vi "Dashboard Main.vi"() -> ()   [LabVIEW 2018]
uses:
  <vilib>/Rock Robotics/WPI/Camera/WPI_CameraExposure Values.ctl
  <vilib>/Rock Robotics/WPI/Camera/WPI_CameraWhite Balance Values.ctl
  <vilib>/Rock Robotics/WPI/Camera/WPI_CameraSettings Read MJPG.ctl
  <vilib>/Rock Robotics/WPI/Camera/WPI_CameraImageSize.ctl
  <vilib>/Utility/miscctls.llb/LVRowAndColumnTypeDef.ctl
  <vilib>/event_ctls.llb/eventvkey.ctl
  <vilib>/Rock Robotics/Network Tables/NT Read Numeric Array.vi
  <vilib>/Rock Robotics/WPI/Dashboard/WPI_DashboardLogging Global.vi
  Dashboard globals.vi
  <vilib>/vision/NI_Vision_Development_Module.lvlib
panel:
  in  "Camera Settings Right":T1={"Frame Rate"=30, "Compression"=30, "Size"=1, "DB Camera Config"=FALSE} {"Frame Rate" scale=1.0..30.0; "Compression" scale=100.0..-1.0; "Size" items=["640x480", "320x240", "160x120"]}
  in  "Camera Name Right":string(combo)="No Camera Selection"
  out "Camera Perf":string
  in  "Camera Settings":T1={"Frame Rate"=30, "Compression"=30, "Size"=1, "DB Camera Config"=FALSE} {"Frame Rate" scale=1.0..30.0; "Compression" scale=100.0..-1.0; "Size" items=["640x480", "320x240", "160x120"]}
  in  "TCP":refnum<k5>
  in  "Rec Mode":enum32{"Stop", "Record", "Playback"}(radio)
  out "Robot IP":string
  out "Image Message":string="Timeout in Camera Communications"
  in  "Dashboard Tab":T2(tab)=enum."Custom"
  in  "Select Auto":string(combo)="Select Autonomous ..."
  out "NT Connection":bool
  out "MotorChart R":cluster{"Numeric":dbl, "Numeric":dbl}(graph)
  out "MotorChart L":cluster{"Numeric":dbl, "Numeric":dbl}(graph)
  out "MotorSliders R":cluster{"MotorSlide1":dbl, "MotorSlide2":dbl} {"MotorSlide2" scale=-1.0..1.0 scale format="%#_2e"; "MotorSlide1" scale=-1.0..1.0 scale format="%#_2e"}
  out "MotorSliders L":cluster{"MotorSlide1":dbl, "MotorSlide2":dbl} {"MotorSlide2" scale=-1.0..1.0 scale format="%#_2e"; "MotorSlide1" scale=-1.0..1.0 scale format="%#_2e"}
  out "Gyro":dbl(knob) scale=0.0..360.0
  out "JS1 Z":dbl(slide) scale=-1.0..1.0 scale format="%#_2e"
  out "JS1 Graph":cluster{"X":dbl, "Y":dbl}[](graph)
  out "JS1 Buttons":T3
  out "JS2 Z":dbl(slide) scale=-1.0..1.0 scale format="%#_2e"
  out "JS2 Graph":cluster{"X":dbl, "Y":dbl}[](graph)
  out "JS2 Buttons":T3
  out "Mode":T4(ring)=enum."Auto Disabled"
  out "Right Camera Perf":cluster{"Bandwidth (Mbps)":dbl, "FPS":dbl}
  out "Camera Image Right":T5(plugin-control)
  in  "DB/String 9":string
  in  "DB/String 8":string
  in  "DB/String 7":string
  in  "DB/String 6":string
  in  "DB/String 5":string
  in  "DB/String 4":string
  in  "DB/String 3":string
  in  "DB/String 2":string
  in  "DB/String 1":string
  in  "DB/String 0":string
  in  "DB/Slider 0":dbl(slide) scale=0.0..5.0
  in  "DB/Slider 1":dbl(slide) scale=0.0..5.0
  in  "DB/Slider 2":dbl(slide) scale=0.0..5.0
  in  "DB/Slider 3":dbl(slide) scale=0.0..5.0
  out "DB/LED 3":bool
  out "DB/LED 2":bool
  out "DB/LED 1":bool
  out "DB/LED 0":bool
  in  "DB/Button 3":bool
  in  "DB/Button 2":bool
  in  "DB/Button 1":bool
  in  "DB/Button 0":bool caption="New Name"
  in  "Desired Target":T6(radio)=enum."Ship Right"
  in  "Enable Vision\nProcessing":bool
  in  "Test Slider":dbl(slide) scale=0.0..100.0 scale format="%#_3g"
  in  "On/Off":bool caption="Solenoid"
  in  "Test Name":u16(ring) items=["Select the test to run..."]
  in  "Test Tree":string(tree)
  in  "Motor":cluster{"Value":dbl, "Enable":bool} {"Value" scale=-1.0..1.0 scale format="%#_3g"}
  out "Progress":T7 {"Test Progress" scale=0.0..100.0}
  in  "Rev/Fwd":cluster{"Forward":bool, "Reverse":bool}
  in  "Test Ring":u16(ring) items=["Monochrome", "Color"]
  out "Cmd Status":string
  in  "Execute Command":bool
  in  "Command Params":string[][](table)
  in  "Command Selection":i32(listbox)
  in  "CheckList":i32(listbox)
  out "Tree":string(tree)
  out "Camera Image":T5(plugin-control)
  out "Background":bool
  in  "Camera Name":string(combo)="No Camera Selection"
  # "HW"
  # "HW"
  # "Joysticks"
  # "Drive Motors"
  # "Front"
  # "Right"
  # "Left"
  # "Back"
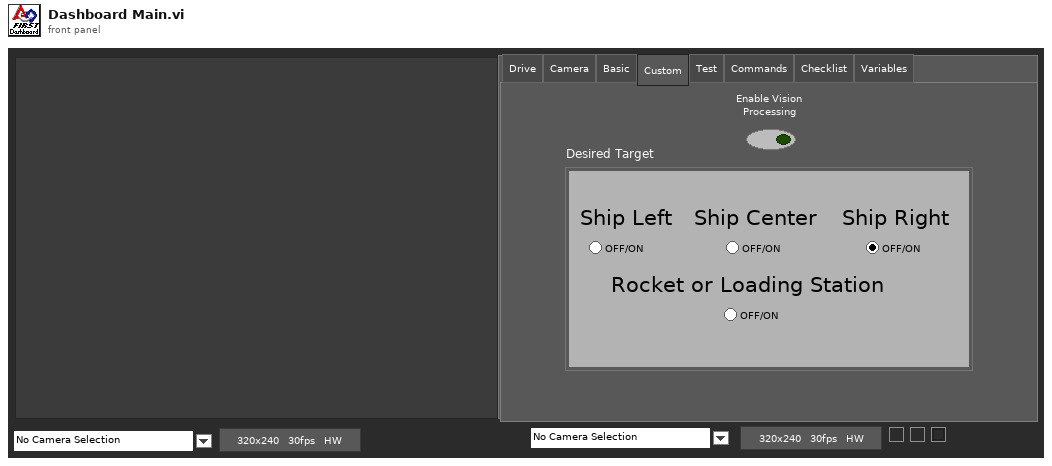
[diagram p1: front panel]
types:
  T1 = cluster{"Frame Rate":i32, "Compression":i32, "Size":u16, "DB Camera Config":bool}
  T2 = enum32{"Drive", "Camera", "Basic", "Custom", "Test", "Commands", "Checklist", "Variables"}
  T3 = cluster{bool, bool, bool, bool, bool, bool, bool, bool, bool, bool, bool, bool}
  T4 = enum8{"Tele-Op Disabled", "Tele-Op Enabled", "Auto Disabled", "Auto Enabled", "Test Disabled", "Test Enabled", "Disconnected", "No Code", "E-Stop"}
  T5 = typedef "IMAQ Image.ctl" = refnum<image>
  T6 = enum32{"Ship Left", "Ship Center", "Ship Right", "Rocket or Loading Station"}
  T7 = cluster{"Test Progress":u8, "Test Progress Text":string}
  T8 = cluster{"Save Path":path, "Interval (s)":dbl, "Keep":i32}
  T9 = typedef "Image Type" = u32
  T10 = cluster{"IDs":cluster{"RPC field ID":u16, "Unique ID":u16}, "String":string}
  T11 = cluster{"Camera Image":refnum<vi>, "Dashboard Tab":refnum<vi>, "Background":refnum<vi>, "Rec Mode":refnum<vi>, "Test Slider":refnum<vi>, "On/Off ":refnum<vi>, "Test Ring":refnum<vi>, "Rev/Fwd":refnum<vi>, "Test Name":refnum<vi>, "Motor":refnum<vi>, "Progress":refnum<vi>, "CheckList":refnum<vi>, "Tree":refnum<vi>, "Test Tree":refnum<vi>, "Command Params":refnum<vi>, "Command Selection":refnum<vi>, "Execute Command":refnum<vi>, "Cmd Status":refnum<vi>, "Camera Settings":refnum<vi>, "Camera Name":refnum<vi>, "Camera Perf":refnum<vi>, "Camera Settings Right":refnum<vi>, "Camera Name Right":refnum<vi>, "Camera Image Right":refnum<vi>}
  T12 = typedef "WPI_CameraSettings Read MJPG.ctl" = cluster{"fps":i32, "compression":i32, "Image Size":T13, "Config Shown":bool}
  T13 = typedef "WPI_CameraImageSize.ctl" = enum16{"640x480", "320x240", "160x120", "Custom"}
  T14 = typedef "WPI_CameraExposure Values.ctl" = enum16{"Auto", "Flicker-free 50 Hz", "Flicker-free 60 Hz", "Hold current", "Custom"}
  T15 = typedef "WPI_CameraWhite Balance Values.ctl" = enum16{"Auto", "Fixed indoor", "Fixed outdoor 1", "Fixed outdoor 2", "Fixed fluorescent 1", "Fixed fluorescent 2", "Hold current", "Custom"}
  T16 = cluster{"Exposure":T14, "Exposure (%)":dbl, "Brightness":i32, "White Balance":T15, "Color Temp (K)":dbl}
  T17 = cluster{"Global Rectangle":i32[], "Contours":cluster{"Contour Type":u32, "ROI Type":u32, "Points":i32[]}[]}
  T18 = cluster{"Camera Name":string, string, "Saved DB Images Info":cluster{"Save Path":path, "Interval (s)":dbl, "Keep":i32}}
  T19 = cluster{"Corners":cluster{"X":sgl, "Y":sgl}[], "Orientation (degrees)":dbl, "Width":dbl, "Height":dbl, "Score":dbl}[]
  T20 = cluster{"Camera Name Right":string, string, "Saved DB Images Info":cluster{"Save Path":path, "Interval (s)":dbl, "Keep":i32}}
  T21 = cluster{"Error Strings":string, "Disable Counts":cluster{u16, u16}, "Rail Faults":cluster{u16, u16, u16}, "Robot IP":string, "DB Mode":u8, "Event Info":cluster{"Name":string, "Type":u8, "Number":u16, "Replay":u8}}
  T22 = cluster{"Storage":cluster{"Disk Free":u64, "RAM Block":u32, "RAM free":u32}, "CPU Utilization":cluster{"CPU % ISR":sgl, "CPU % Time Crit":sgl, "CPU % Timed Str":sgl, "CPU % High":sgl, "CPU % Above":sgl, "CPU % Normal":sgl, "CPU % Low":sgl}, "CAN":cluster{"% Bus Utilization":sgl, "Bus Off Cnt":u32, "TX_FIFO Full Cnt":u32, "Receive Error Cnt":u8, "Transmit Error Cnt":u8}, "HID":cluster{"HID Outputs":u32, "Rumble Low":u16, "Rumble High":u16}[]}
  T23 = cluster{"Status bits":cluster{"Test Mode":bool, "Autonomous":bool, "Enabled":bool, "Code Start":bool, "Brownout":bool, "Reserved 2":bool, "Reserved 3":bool, "E-Stop":bool}, "Code Trace":cluster{"Disabled":bool, "TeleOp":bool, "Auto":bool, "Test":bool}, "Controller Type":enum16{"unknown", "cRIO", "roboRio"}, "Code?":enum16{"unknown", "noCode", "code"}, "Battery V":dbl}
  T24 = cluster{"Control Bits":cluster{"TestMode":bool, "Autonomous":bool, "Enabled":bool, "FMS Present":bool, bool, bool, bool, "E-Stop":bool}, "Team Station ":u8, "Countdown":sgl, "Joystick Values":cluster{"Axes":dbl[], "Buttons":bool[], "POVs":i16[]}[]}
  T25 = cluster{"Axes":dbl[], "Buttons":bool[], "POVs":i16[]}[]
  T26 = cluster{"Axes":dbl[], "Buttons":bool[], "POVs":i16[]}
  T27 = cluster{"Buttons[0]":bool, "Buttons[1]":bool, "Buttons[2]":bool, "Buttons[3]":bool, "Buttons[4]":bool, "Buttons[5]":bool, "Buttons[6]":bool, "Buttons[7]":bool, "Buttons[8]":bool, "Buttons[9]":bool, "Buttons[10]":bool, "Buttons[11]":bool}
  T28 = cluster{"Operation":enum16{"Update", "Clear"}, "Color Box":u32}[]
  T29 = typedef "eventvkey.ctl" = enum16{"ASCII", "Enter", "Return", "Shift", "Ctrl", "Alt", "Cmd", "Opt", "Caps", "NumLock", "Clear", "Break", "Up", "Down", "Left", "Right", "Insert", "Delete", "Home", "End", "PageUp", "PageDown", "Escape", "Help", "Pause", "ScrollLock", "F1", "F2", "F3", "F4", "F5", "F6", "F7", "F8", "F9", "F10", "F11", "F12", "F13", "F14", "F15", "F16", "F17", "F18", "F19", "F20", "F21", "F22", "F23", "F24", "Play", "VolumeUp", "VolumeDown", "Mute", "Two Byte Char"}
  T30 = cluster{"Image Size":bool, "Image Type":bool, "Pixel Value":bool, "ROI Information":bool, "Zoom Factor":bool}
  T31 = cluster{"Operation":enum16{"Update", "Clear"}, "Color Box":u32}
  T32 = typedef "LVRowAndColumnTypeDef.ctl" = cluster{"Row":i32, "Column":i32}
  T33 = cluster{"Shift":bool, "Ctrl":bool, "Alt":bool, "Cmd":bool, "Opt":bool}
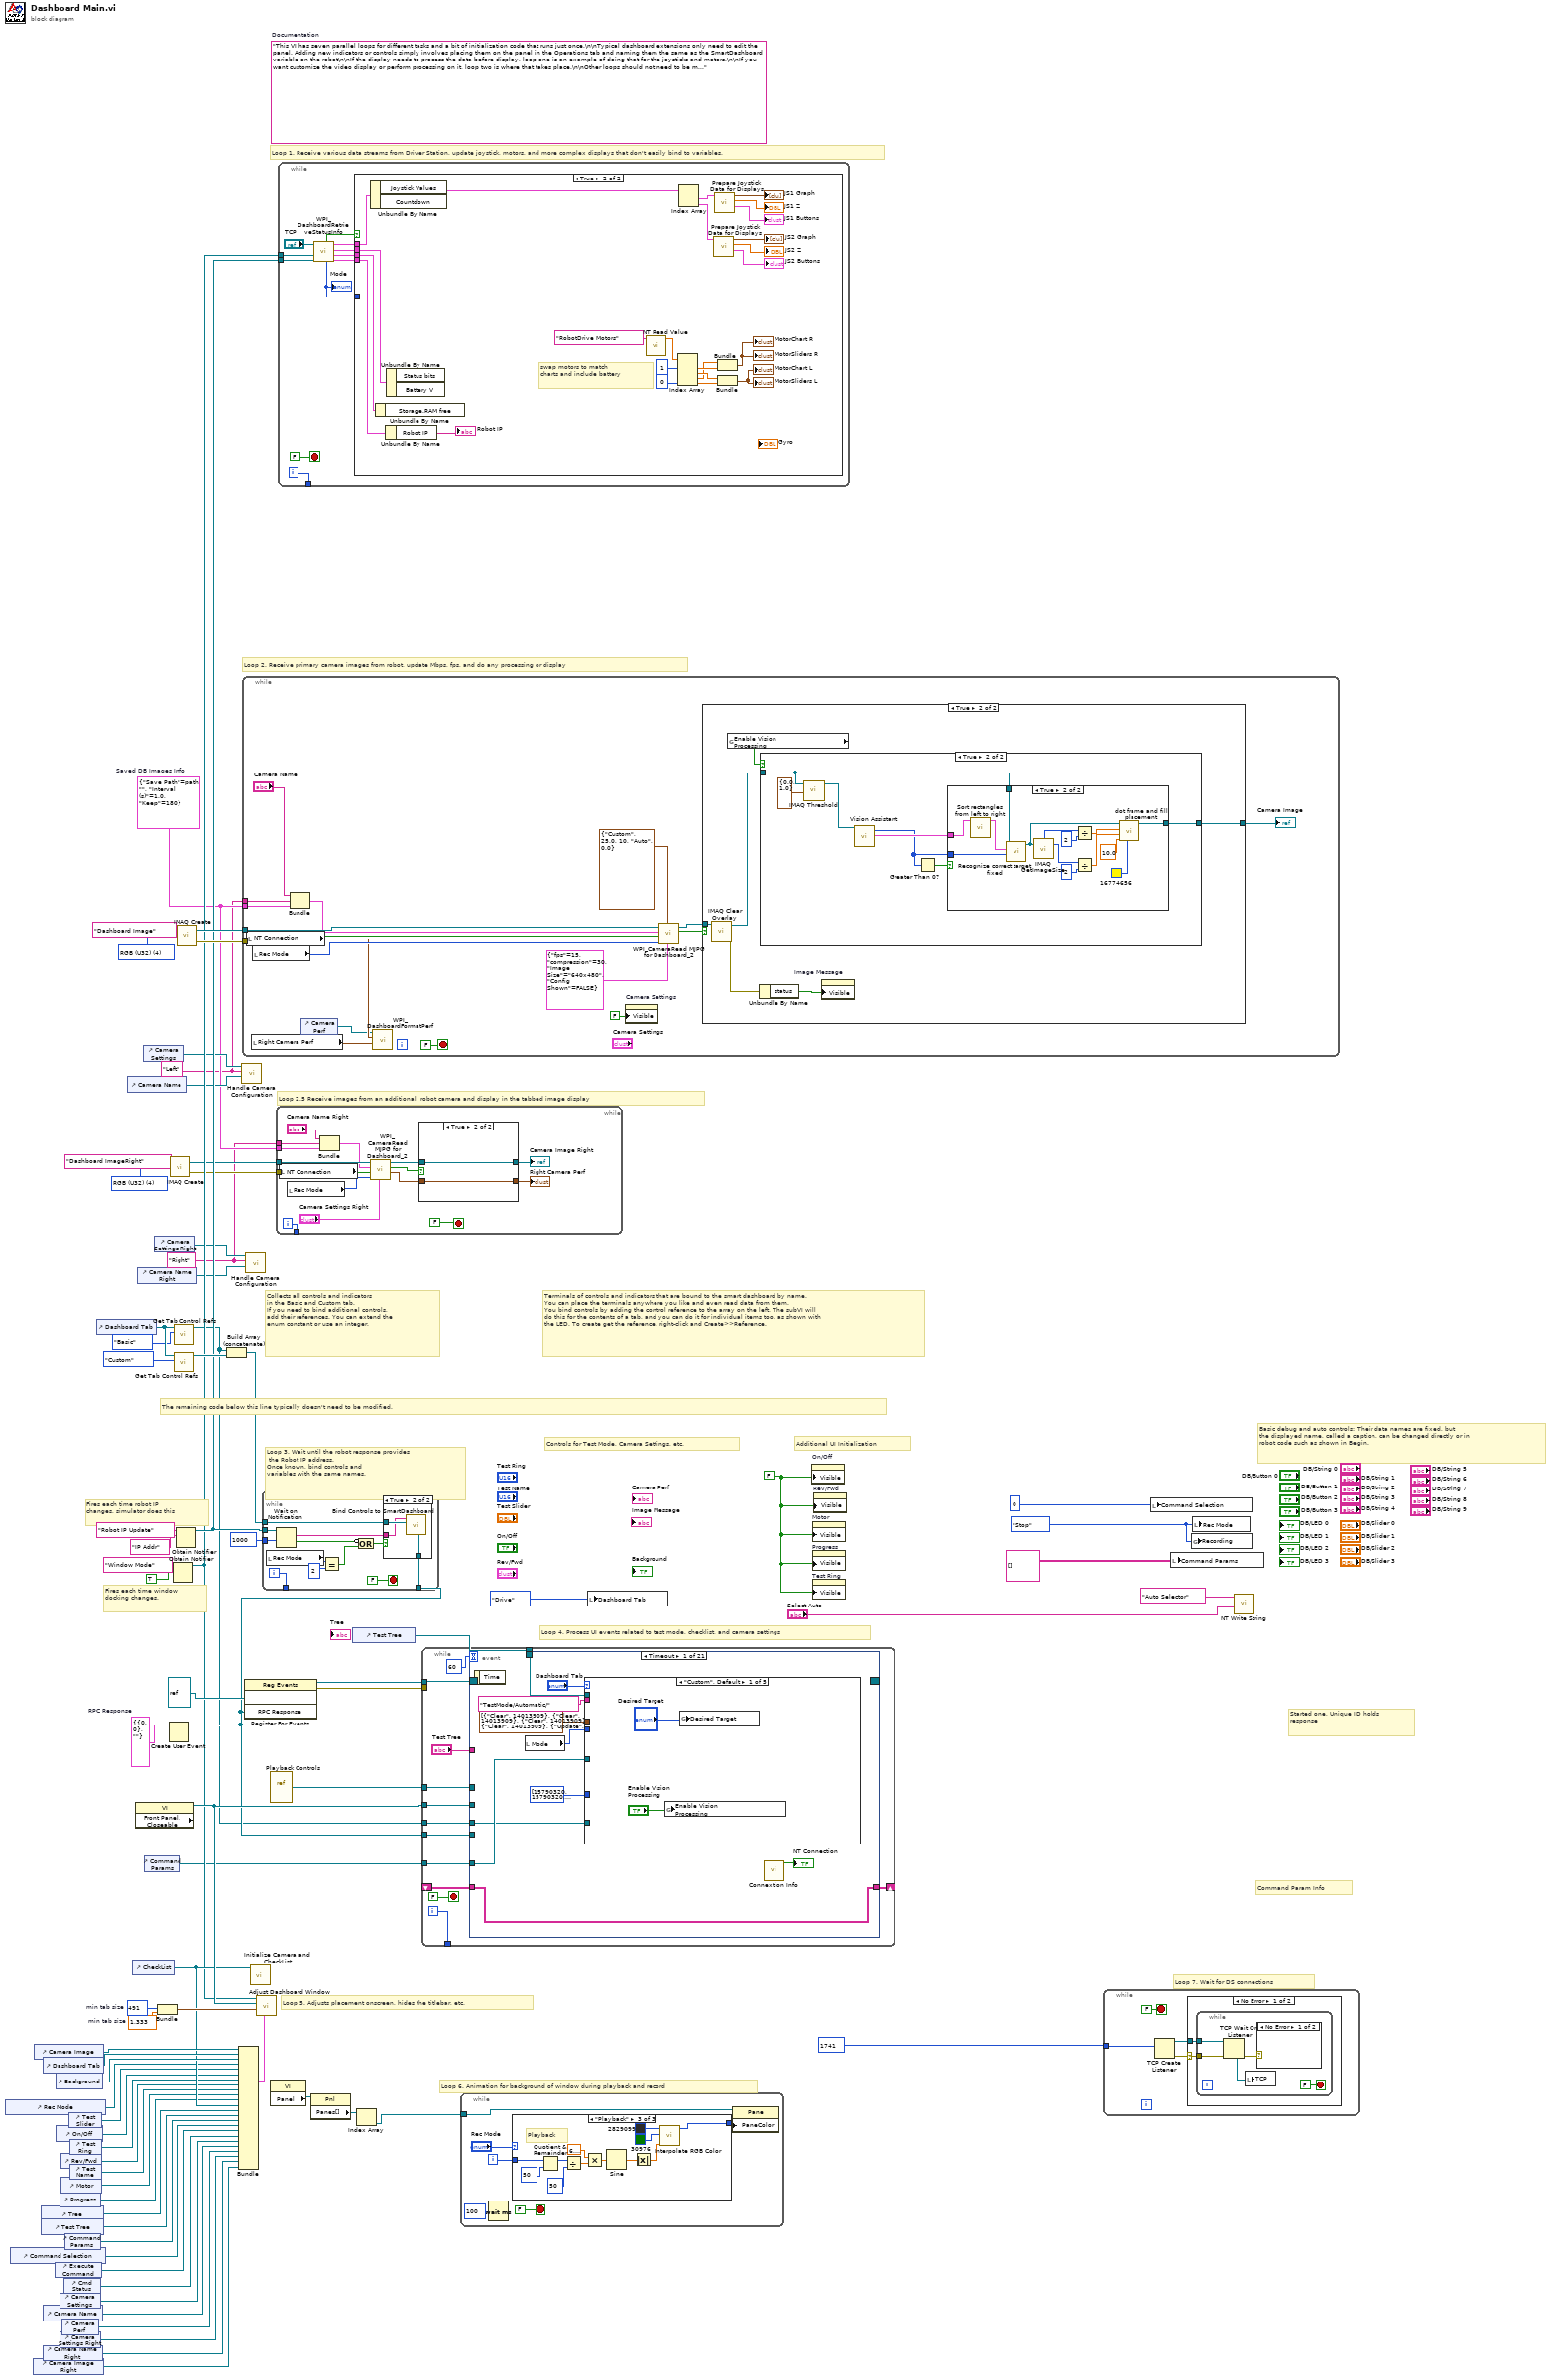
[diagram p0: block diagram]
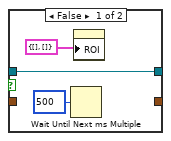
[diagram p2: hidden frame]
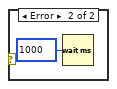
[diagram p3: hidden frame]
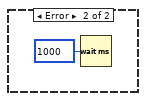
[diagram p4: hidden frame]
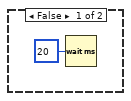
[diagram p5: hidden frame]
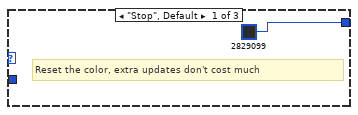
[diagram p6: hidden frame]
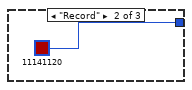
[diagram p7: hidden frame]
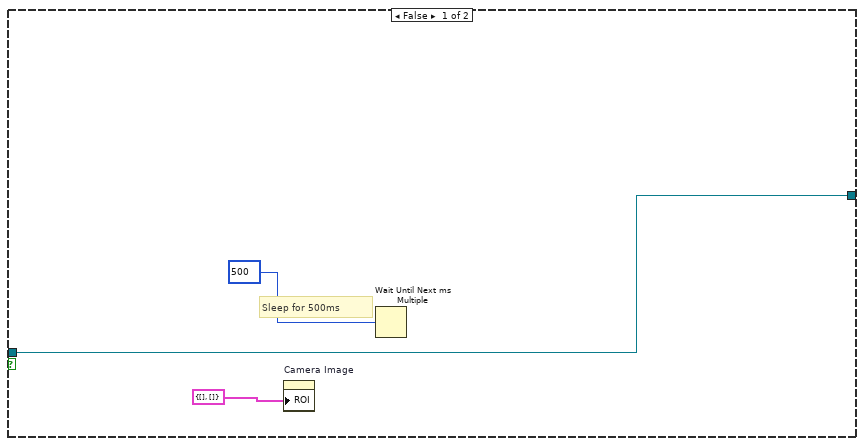
[diagram p9: hidden frame]
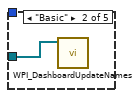
[diagram p12: hidden frame]
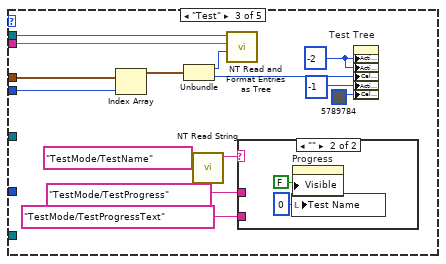
[diagram p13: hidden frame]
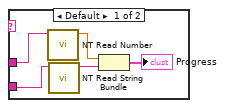
[diagram p14: hidden frame]
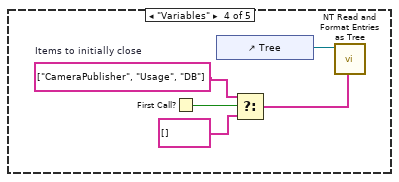
[diagram p15: hidden frame]
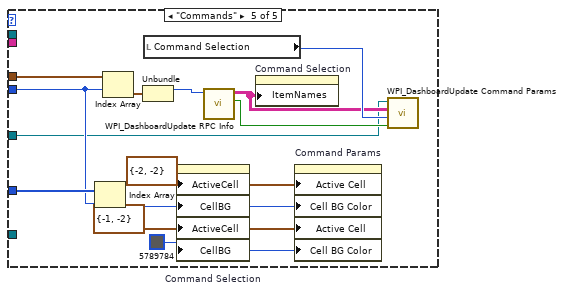
[diagram p16: hidden frame]
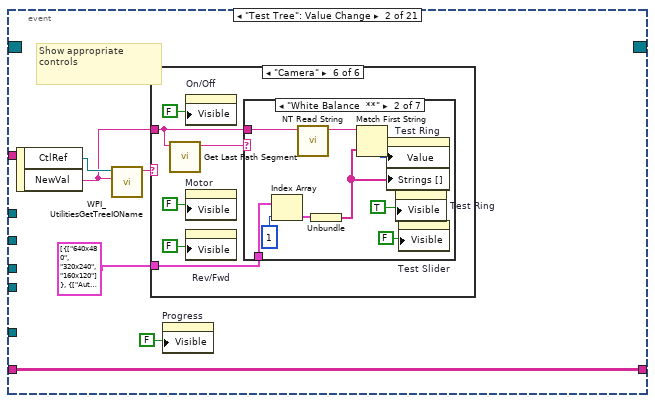
[diagram p17: hidden frame]
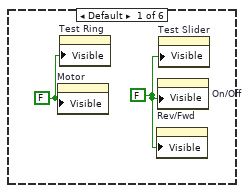
[diagram p18: hidden frame]
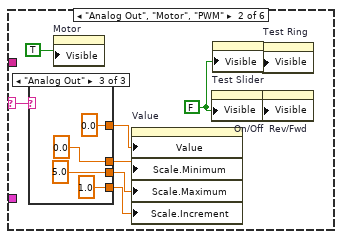
[diagram p19: hidden frame]
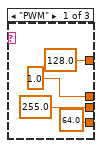
[diagram p20: hidden frame]
diagram:
  w3 = T8 {"Save Path"=path "", "Interval (s)"=1.0, "Keep"=180}  # Saved DB Images Info
  w2 = "Right"
  w1 = "Left"
  w13 = T9 4 items=["Grayscale (U8)", "Grayscale (I16)", "Grayscale (SGL)", "Complex (CSG)", "RGB (U32)", "HSL (U32)", "RGB (U64)"] ("Image Type")
  w29 = T10 {"IDs"={"RPC field ID"=0, "Unique ID"=0}, "String"=""}  # RPC Response
  w52 = 491  # min tab size
  w51 = 1.333  # min tab size
  w59 = enum32{"Stop", "Record", "Playback"}."Stop" ("Rec Mode")
  w36 = FALSE ("Visible")
  (unwired) "This VI has seven parallel loops for different tasks and a bit of initialization code that runs just once.\n\nTypical dashboard extensions only need to edit the panel. Adding new indicators or controls simply involves placing them on the panel in the Operations tab and naming them the same as the SmartDashboard variable on the robot\n\nIf the display needs to process the data before display, loop one is an example of doing that for the joysticks and motors.\n\nIf you want customize the video display or perform processing on it, loop two is where that takes place.\n\nOther loops should not need to be modified. They are pretty standard, and document the task they perform."  # Documentation
  w76 = T9 4 items=["Grayscale (U8)", "Grayscale (I16)", "Grayscale (SGL)", "Complex (CSG)", "RGB (U32)", "HSL (U32)", "RGB (U64)"] ("Image Type")
  # "Loop 2.5 Receive images from an additional  robot camera and display in the tabbed image display"
  # "Command Param Info"
  # "Started one, Unique ID holds\nresponse"
  # "Loop 7. Wait for DS connections"
  # "Basic debug and auto controls: Their data names are fixed, but\nthe displayed name, called a caption, can be changed directly or in\nrobot code such as shown in Begin."
  # "Controls for Test Mode, Camera Settings, etc."
  # "Additional UI Initialization"
  # "Loop 6. Animation for background of window during playback and record"
  # "Fires each time robot IP\nchanges, simulator does this"
  # "Fires each time window\ndocking changes."
  # "Collects all controls and indicators\nin the Basic and Custom tab.\nIf you need to bind additional controls,\nadd their references. You can extend the\nenum constant or use an integer."
  # "The remaining code below this line typically doesn't need to be modified."
  # "Loop 4. Process UI events related to test mode, checklist, and camera settings"
  # "Terminals of controls and indicators that are bound to the smart dashboard by name.\nYou can place the terminals anywhere you like and even read data from them.\nYou bind controls by adding the control reference to the array on the left. The subVI will\ndo this for the contents of a tab, and you can do it for individual items too, as shown with\nthe LED. To create get the reference, right-click and Create>>Reference."
  # "Loop 3. Wait until the robot response provides\n the Robot IP address.\nOnce known, bind controls and\nvariables with the same names."
  # "Loop 5. Adjusts placement onscreen, hides the titlebar, etc."
  # "Loop 1. Receive various data streams from Driver Station, update joystick, motors, and more complex displays that don't easily bind to variables."
  # "Loop 2. Receive primary camera images from robot, update Mbps, fps, and do any processing or display"
  n1 = control-ref of="Rec Mode"() -> (w42:refnum<vi>)
  n2 = control-ref of="Command Selection"() -> (w28:refnum<vi>)
  n3 = control-ref of="Camera Image Right"() -> (w6:refnum<vi>)
  n4 = control-ref of="Camera Image"() -> (w54:refnum<vi>)
  n5 = control-ref of="Tree"() -> (w46:refnum<vi>)
  n6 = control-ref of="Test Tree"() -> (w45:refnum<vi>)
  n7 = control-ref of="Camera Name"() -> (w19:refnum<vi>)
  n8 = control-ref of="Camera Name Right"() -> (w7:refnum<vi>)
  n9 = control-ref of="Dashboard Tab"() -> (w53:refnum<vi>)
  n10 = control-ref of="Execute Command"() -> (w30:refnum<vi>)
  n11 = control-ref of="Background"() -> (w49:refnum<vi>)
  n12 = control-ref of="On/Off"() -> (w40:refnum<vi>)
  n13 = control-ref of="Progress"() -> (w37:refnum<vi>)
  n14 = control-ref of="Camera Settings"() -> (w20:refnum<vi>)
  n15 = control-ref of="Camera Settings Right"() -> (w8:refnum<vi>)
  n16 = control-ref of="Rev/Fwd"() -> (w38:refnum<vi>)
  n17 = control-ref of="Motor"() -> (w43:refnum<vi>)
  n18 = control-ref of="Camera Perf"() -> (w18:refnum<vi>)
  n19 = control-ref of="Cmd Status"() -> (w24:refnum<vi>)
  n20 = control-ref of="Command Params"() -> (w31:refnum<vi>)
  n21 = control-ref of="Test Slider"() -> (w41:refnum<vi>)
  n22 = control-ref of="Test Ring"() -> (w39:refnum<vi>)
  n23 = control-ref of="Test Name"() -> (w44:refnum<vi>)
  n24 = control-ref of="Dashboard Tab"() -> (w57:refnum<vi>)
  n25 = control-ref of="Camera Name"() -> (w21:refnum<vi>)
  n26 = control-ref of="CheckList"() -> (w47:refnum<vi>)
  n27 = property class="VI" props=["Front Panel.Closeable"]() -> (reference out=w58:refnum<vi>)  [unwired: 2 in, 2 out]
  n28 = control-ref of="Camera Name Right"() -> (w9:refnum<vi>)
  n29 = control-ref of="Camera Settings"() -> (w22:refnum<vi>)
  n30 = control-ref of="Command Params"() -> (w23:refnum<vi>)
  n31 = control-ref of="Camera Settings Right"() -> (w10:refnum<vi>)
  n32 = Bundle("min tab size"=w52, "min tab size"=w51) -> (w50:cluster{"min tab size":i32, "min tab size":dbl})  [unwired: 1 in]
  n33 = Create User Event(user event datatype=w29) -> (user event=w25:refnum<user-event>)  [unwired: 1 in, 1 out]
  n34 = call "IMAQ Create"("Image Name"="Dashboard ImageRight", "Image Type"=w13) -> ("New Image"=w12:T5, "error out"=w11:errorcluster)  [unwired: 2 in, 1 out]
  n35 = Obtain Notifier(name (unnamed)="Window Mode", notification data type=TRUE) -> (notifier out=w34:refnum<notifier>)  [unwired: 2 in, 2 out]
  n36 = call <vilib>:"Get Tab Control Refs.vi"("Page Index"=T2."Basic" ("Dashboard Tab"), "TabControl in"=w57) -> ("ControlsOnPage"=w17:refnum<vi>[])  [unwired: 9 in]
  n37 = call <vilib>:"Get Tab Control Refs.vi"("Page Index"=T2."Custom" ("Dashboard Tab"), "TabControl in"=w57) -> ("ControlsOnPage"=w56:refnum<vi>[])  [unwired: 9 in]
  n38 = Obtain Notifier(name (unnamed)="Robot IP Update", notification data type="IP Addr" ("name (unnamed)")) -> (notifier out=w35:refnum<notifier>)  [unwired: 2 in, 2 out]
  n39 = call "IMAQ Create"("Image Name"="Dashboard Image", "Image Type"=w76) -> ("New Image"=w74:T5, "error out"=w73:errorcluster)  [unwired: 2 in, 1 out]
  n40 = Build Array (concatenate)(w17, w56) -> (w55:refnum<vi>[])
  n41 = Bundle("Camera Image"=w54, "Dashboard Tab"=w53, "Background"=w49, "Rec Mode"=w42, "Test Slider"=w41, "On/Off"=w40, "Test Ring"=w39, "Rev/Fwd"=w38, "Test Name"=w44, "Motor"=w43, "Progress"=w37, "CheckList"=w47, "Tree"=w46, "Test Tree"=w45, "Command Params"=w31, "Command Selection"=w28, "Execute Command"=w30, "Cmd Status"=w24, "Camera Settings"=w20, "Camera Name"=w19, "Camera Perf"=w18, "Camera Settings Right"=w8, "Camera Name Right"=w7, "Camera Image Right"=w6) -> (w48:T11)  [unwired: 1 in]
  n42 = call "Handle Camera Configuration.vi"("CameraNameRef"=w21, "Display Name"=w1, "ClusterRef"=w22) -> ()  [unwired: 9 in]
  n43 = while {
    tunnel: w74 -> [w92]
    tunnel: w73 -> [_]
    tunnel: w3 -> [w86]
    tunnel: w1 -> [w83]
    stop <- FALSE stop-if-true
    n44 = local read "NT Connection"() -> (w87:bool)
    n45 = local read "Right Camera Perf"() -> (w81:cluster{"Bandwidth (Mbps)":dbl, "FPS":dbl})
    n46 = local read "Rec Mode"() -> (w89:enum32{"Stop", "Record", "Playback"})
    n47 = Bundle("Camera Name"="Camera Name", w83, "Saved DB Images Info"=w86) -> (w85:T18)  [unwired: 1 in]
    n48 = control-ref of="Camera Perf"() -> (w80:refnum<vi>)
    n49 = property on="Camera Settings" class="Clust (strict)"("Visible"=FALSE) -> ()  [unwired: 2 in, 2 out]
    n50 = call <vilib>:"WPI_CameraRead MJPG for Dashboard_2.vi"("Camera Settings"=T12 {"fps"=15, "compression"=30, "Image Size"=enum."640x480", "Config Shown"=FALSE}, "Camera Settings 2"=T16 {"Exposure"=enum."Custom", "Exposure (%)"=25.0, "Brightness"=10, "White Balance"=enum."Auto", "Color Temp (K)"=0.0}, "Rec Mode"=w89, "NT Connection"=w87, "Capture Info"=w85, "Image in"=w92) -> ("perf info"=w82:cluster{"Bandwidth (Mbps)":dbl, "fps":dbl}, "Active"=w90:bool, "Image\\ out"=w91:T5)  [unwired: 3 in]
    n51 = call <vilib>:"WPI_DashboardFormatPerf.vi"("Right Camera Perf"=w81, "Performance"=w82, "String in"=w80) -> ()  [unwired: 9 in]
    n52 = case shown="True" w90 {
      tunnel: w91 -> [w95 w100]
      tunnel: [w95 w98] -> w88
      frame False {
        # "Sleep for 500ms"
        n53 = property on="Camera Image" class="ImageControl"("ROI"=T17 {"Global Rectangle"=[], "Contours"=[]}) -> ()  [unwired: 2 in, 2 out]
        n54 = Wait Until Next ms Multiple(millisecond multiple=u32 500) -> ()  [unwired: 1 out]
      }
      frame True {
        n55 = call "IMAQ Clear Overlay"("Image"=w100) -> ("error out"=w101:errorcluster, "Image Out"=w99:T5)  [unwired: 2 in, 7 out]
        n56 = global read "Dashboard globals.vi" "Enable Vision\nProcessing"() -> (w97:bool)
        n57 = Unbundle By Name(w101) -> ("status"=w102:bool)
        n58 = case shown="True" w97 {
          tunnel: w99 -> [w103 w109]
          tunnel: [w103 w104] -> w98
          frame False {
          }
          frame True {
            n59 = call "IMAQ Threshold"("Range"=cluster{"Lower value":sgl, "Upper value":sgl} {"Lower value"=0.0, "Upper value"=1.0}, "Image Src"=w109) -> ("Image Dst Out"=w108:T5)  [unwired: 8 in, 1 out]
            n60 = call "Vision Assistant"("Image In"=w108) -> ("Number of Matches (Shape Detection 1)"=w105:i32, "Rectangles Calibrated (Shape Detection 1)"=w106:T19)  [unwired: 23 in, 2 out]
            n61 = Greater Than 0?(x=w105) -> (x > 0?=w107:bool)
            n62 = case shown="True" w107 {
              tunnel: w109 -> [w111 w125]
              tunnel: w106 -> [_ w124]
              tunnel: w105 -> [_ w123]
              tunnel: [w111 w113] -> w104
              frame False {
              }
              frame True {
                n63 = call "Sort rectangles from left to right.vi"("Rectangles (Calibrated) IN"=w124) -> ("Rectangles (Calibrated) OUT"=w122:T19)  [unwired: 10 in]
                n64 = call "Recognize correct target fixed.vi"("# rectangles"=w123, "Rectangles (Calibrated)"=w122, "Image"=w125) -> ("Image Out"=w121:T5)  [unwired: 8 in]
                n65 = call "IMAQ GetImageSize"("Image"=w121) -> ("Y Resolution"=w119:i32, "X Resolution"=w120:i32)  [unwired: 3 in, 1 out]
                n66 = Divide(x=w120, y=2) -> (x/y=w117:dbl)
                n67 = Divide(x=w119, y=2) -> (x/y=w118:dbl)
                n68 = call "dot frame and fill placement.vi"("Color"=u32 16774656, "size"=sgl 10.0, "y coordinate"=w118, "x coordinate"=w117, "Image"=w121) -> ("Image Out"=w113:T5)  [unwired: 6 in]
              }
            }
          }
        }
        n69 = property on="Image Message" class="Str"("Visible"=w102) -> ()  [unwired: 2 in, 2 out]
      }
    }
    "Camera Image" <- w88
  }
  n70 = register-events(refnum<vi> refnum, w25) -> (reference out=w63:refnum<event-registration>, error out=w62:errorcluster)  [unwired: 2 in]
  n71 = call "Handle Camera Configuration.vi"("CameraNameRef"=w9, "Display Name"=w2, "ClusterRef"=w10) -> ()  [unwired: 9 in]
  n72 = call "Initialize Camera and CheckList.vi"("ListBox in"=w47) -> ()  [unwired: 11 in]
  n73 = call "Adjust Dashboard Window.vi"("Sizing Refnums"=w48, "Size Constraints"=w50, "VI"=w58, "WIn Mode"=w34) -> ()  [unwired: 8 in]
  n74 = while {
    tunnel: w55 -> [w137]
    tunnel: w35 -> [w135]
    tunnel: [w133] -> _
    tunnel: u32 1000 ("milliseconds to wait") -> [w132]
    tunnel: w25 -> [w126]
    i -> [w133]
    stop <- FALSE stop-if-true
    n75 = local read "Rec Mode"() -> (w128:enum32{"Stop", "Record", "Playback"})
    n76 = Wait on Notification(notifier=w135, timeout in ms (-1)=w132) -> (notification=w134:string, timed out?=w130:bool)  [unwired: 2 in, 2 out]
    n77 = Equal?(x=w128, y=u16 2 ("Rec Mode")) -> (x = y?=w129:bool)
    n78 = Compound Arithmetic op=OR(invert w130, w129) -> (w131:bool)
    n79 = case shown="True" w131 {
      tunnel: w137 -> [_ w140]
      tunnel: w134 -> [_ w139]
      tunnel: w126 -> [_ w138]
      frame False {
      }
      frame True {
        n80 = call <vilib>:"Bind Controls to SmartDashboard.vi"("RPC ref"=w138, "Bound Control Refs"=w140, "Server IP Address"=w139) -> ()  [unwired: 9 in]
      }
    }
  }
  n81 = vi-ref "Playback Controls.vi"() -> (w64:refnum<vi>)
  n82 = property class="VI"() -> ("Panel"=w66:refnum<vi>)  [unwired: 2 in, 2 out]
  n83 = while {
    tunnel: w12 -> [w155]
    tunnel: w11 -> [_]
    tunnel: [w150] -> _
    tunnel: w3 -> [w146]
    tunnel: w2 -> [w143]
    i -> [w150]
    stop <- FALSE stop-if-true
    n84 = local read "NT Connection"() -> (w147:bool)
    n85 = local read "Rec Mode"() -> (w154:enum32{"Stop", "Record", "Playback"})
    n86 = Bundle("Camera Name Right"="Camera Name Right", w143, "Saved DB Images Info"=w146) -> (w145:T20)  [unwired: 1 in]
    n87 = call <vilib>:"WPI_CameraRead MJPG for Dashboard_2.vi"("Camera Settings"="Camera Settings Right", "Rec Mode"=w154, "NT Connection"=w147, "Capture Info"=w145, "Image in"=w155) -> ("perf info"=w141:cluster{"Bandwidth (Mbps)":dbl, "fps":dbl}, "Active"=w149:bool, "Image\\ out"=w152:T5)  [unwired: 4 in]
    n88 = case shown="True" w149 {
      tunnel: w152 -> [w157 w160]
      tunnel: [w157 w160] -> w148
      tunnel: [_ w159] -> w142
      tunnel: w141 -> [_ w159]
      frame False {
        n89 = Wait Until Next ms Multiple(millisecond multiple=u32 500) -> ()  [unwired: 1 out]
        n90 = property on="Camera Image Right" class="ImageControl"("ROI"=T17 {"Global Rectangle"=[], "Contours"=[]}) -> ()  [unwired: 2 in, 2 out]
      }
      frame True {
      }
    }
    "Camera Image Right" <- w148
    "Right Camera Perf" <- w142
  }
  n91 = while {
    tunnel: [w170] -> _
    tunnel: w35 -> [w164]
    tunnel: w34 -> [w161]
    i -> [w170]
    stop <- FALSE stop-if-true
    n92 = call <vilib>:"WPI_DashboardRetrieveStatusInfo.vi"("Binding Refnum"=w164, "Window Mode Notifier"=w161, "TCP Cnx"="TCP") -> ("Power and Errors"=w165:T21, "Robot Metrics"=w168:T22, "Status Info"=w169:T23, "Control Info"=w166:T24, "Robot Mode"=w163:T4, "Process?"=w167:bool)  [unwired: 3 in]
    "Mode" <- w163
    n93 = case shown="True" w167 {
      tunnel: w169 -> [_ w196]
      tunnel: w168 -> [_ w195]
      tunnel: w166 -> [_ w194]
      tunnel: w165 -> [_ w193]
      tunnel: w163 -> [_ _]
      frame False {
        n94 = Wait (ms)(milliseconds to wait=u32 20) -> ()  [unwired: 1 out]
      }
      frame True {
        # "swap motors to match\ncharts and include battery"
        n95 = Unbundle By Name(w194) -> ("Joystick Values"=w184:T25)  [unwired: 1 out]
        n96 = Unbundle By Name(w195) -> ()  [unwired: 1 out]
        n97 = Unbundle By Name(w193) -> ("Robot IP"=→"Robot IP":string)
        n98 = Unbundle By Name(w196) -> ()  [unwired: 2 out]
        n99 = call-poly <vilib>:"NT Read Value.vi"("Name"="RobotDrive Motors") -> ("Numeric Array"=w174:dbl[])  [unwired: 9 in, 1 out]
        n100 = Index Array(array=w174, index #1=1, index #4=0) -> (element #1=w188:dbl, element #2=w189:dbl, element #3=w187:dbl, element #4=w192:dbl)  [unwired: 2 in]
        n101 = Index Array(array=w184) -> (element #1=w183:T26, element #2=w179:T26)  [unwired: 2 in]
        n102 = call "Prepare Joystick Data for Displays.vi"("Joystick Values"=w179) -> ("Buttons"=→"JS2 Buttons":T27, "Z Axis"=→"JS2 Z":dbl, "Cartesian Data"=→"JS2 Graph":cluster{"X axis":dbl, "X axis":dbl}[])  [unwired: 8 in]
        n103 = call "Prepare Joystick Data for Displays.vi"("Joystick Values"=w183) -> ("Buttons"=→"JS1 Buttons":T27, "Z Axis"=→"JS1 Z":dbl, "Cartesian Data"=→"JS1 Graph":cluster{"X axis":dbl, "X axis":dbl}[])  [unwired: 8 in]
        n104 = Bundle("Numeric"=w187, "Numeric"=w188) -> (→"MotorChart R" →"MotorSliders R":cluster{"Numeric":dbl, "Numeric":dbl})  [unwired: 1 in]
        n105 = Bundle("Numeric"=w189, "Numeric"=w192) -> (→"MotorChart L" →"MotorSliders L":cluster{"Numeric":dbl, "Numeric":dbl})  [unwired: 1 in]
      }
    }
  }
  n106 = property class="Pnl"(reference=w66) -> ("Panes[]"=w67:refnum<vi>[])  [unwired: 1 in, 2 out]
  n107 = control-ref of="Test Tree"() -> (w68:refnum<vi>)
  n108 = Index Array(array=w67) -> (element=w65:refnum<vi>)  [unwired: 1 in]
  n109 = while {
    tunnel: [w206] -> _
    tunnel: w68 -> [w205]
    tunnel: w64 -> [w204]
    tunnel: w63 -> [w203]
    tunnel: w62 -> [_]
    tunnel: w58 -> [w202]
    tunnel: w25 -> [w201]
    tunnel: w23 -> [w200]
    shift-right: [w199] -> _
    shift-left: _ -> [w198]
    tunnel: w17 -> [w197]
    i -> [w206]
    stop <- FALSE stop-if-true
    n110 = event shown="[0] Timeout" {
      selector: w203 -> [_ _ _ _ _ _ _ _ _ _ _ _ _ _ _ _ _ _ _ _ _]
      dyn-events: [_ _ _ _ _ _ _ _ _ _ _ _ _ _ _ _ w468 _ _ _ _] -> _
      timeout: u32 60 ("milliseconds to wait") -> [_ _ _ _ _ _ _ _ _ _ _ _ _ _ _ _ _ _ _ _ _]
      tunnel: w205 -> [w218 _ _ _ _ _ _ _ _ _ _ _ _ _ _ _ _ _ _ _ _]
      tunnel: "Test Tree" -> [_ _ _ _ _ _ _ _ _ _ _ w435 w443 w445 w449 w457 _ _ _ _ _]
      tunnel: w204 -> [_ _ _ _ _ _ _ _ _ _ _ _ _ _ _ _ w470 _ w488 _ _]
      tunnel: w202 -> [_ _ _ _ _ _ _ _ _ _ _ _ _ _ _ _ w466 _ _ _ _]
      tunnel: w201 -> [_ _ _ _ _ _ _ _ _ _ _ _ _ _ _ _ w464 _ _ _ _]
      tunnel: w200 -> [w213 _ _ _ _ _ w386 _ _ _ _ _ _ _ _ _ _ _ _ _ _]
      tunnel: [w212 w263 w365 w370 w379 w383 w384 w393 w403 w410 w422 w434 w441 w444 w448 w456 w463 w483 w485 w489 w502] -> w199
      tunnel: w198 -> [w212 w263 w365 w370 w379 w383 w384 _ _ w410 w422 w434 w441 w444 w448 w456 w463 w483 w485 w489 w502]
      tunnel: w197 -> [w210 _ _ _ _ _ _ _ _ _ _ _ _ _ _ _ _ _ _ _ _]
      event Timeout {
        n111 = event-data() -> ()  [unwired: 1 in, 1 out]
        n112 = local read "Mode"() -> (w215:T4)
        n113 = case shown="\"Custom\", Default" "Dashboard Tab" {
          tunnel: w218 -> [_ _ w236 _ _]
          tunnel: "TestMode/Automatic/" ("Name Pattern") -> [_ _ w235 _ _]
          tunnel: T28 [{"Operation"=enum."Clear", "Color Box"=14013909}, {"Operation"=enum."Clear", "Color Box"=14013909}, {"Operation"=enum."Clear", "Color Box"=14013909}, {"Operation"=enum."Clear", "Color Box"=14013909}, {"Operation"=enum."Update", "Color Box"=14013909}, {"Operation"=enum."Update", "Color Box"=16777215}, {"Operation"=enum."Clear", "Color Box"=14013909}, {"Operation"=enum."Clear", "Color Box"=14013909}, {"Operation"=enum."Clear", "Color Box"=14013909}] -> [_ _ w228 _ w256]
          tunnel: w215 -> [_ _ w227 _ w255]
          tunnel: u32[] [15790320, 15790320, 15790320, 15790320, 16777215, 16777215, 15790320, 15790320, 15790320] -> [_ _ _ _ w261]
          tunnel: w213 -> [_ _ _ _ w249]
          tunnel: w210 -> [_ w222 _ _ _]
          frame "Custom", Default {
            n114 = global write "Dashboard globals.vi" "Enable Vision\nProcessing"("Enable Vision\nProcessing") -> ()
            n115 = global write "Dashboard globals.vi" "Desired Target"("Desired Target") -> ()
          }
          frame "Basic" {
            n116 = call <vilib>:"WPI_DashboardUpdateNames.vi"("Controls on Tab"=w222) -> ()  [unwired: 11 in]
          }
          frame "Test" {
            w234 = -2 ("Active Item:Row Number")
            n117 = Index Array(array=w228, index=w227) -> (element=w229:T31)
            n118 = Unbundle(w229) -> ("Operation"=w230:enum16{"Update", "Clear"}, "Color Box"=w231:u32)
            n119 = call <vilib>:"NT Read String.vi"("Name"="TestMode/TestName") -> ("String"=w225:string)  [unwired: 9 in, 1 out]
            n120 = call <vilib>:"NT Read and Format Entries as Tree.vi"("Operation"=w230, "Name Pattern"=w235, "Tree Refnum"=w236) -> ()  [unwired: 7 in, 2 out]
            n121 = case shown="\"\"" w225 {
              tunnel: "TestMode/TestProgress" ("Name") -> [w238 _]
              tunnel: "TestMode/TestProgressText" ("Name") -> [w237 _]
              frame Default {
                n122 = call <vilib>:"NT Read Number.vi"("Name"=w238) -> ("Numeric"=w239:dbl)  [unwired: 9 in, 1 out]
                n123 = call <vilib>:"NT Read String.vi"("Name"=w237) -> ("String"=w240:string)  [unwired: 9 in, 1 out]
                n124 = Bundle("Numeric"=w239, "String"=w240) -> (→"Progress":cluster{"Numeric":dbl, "String":string})  [unwired: 1 in]
              }
              frame "" {
                n125 = local write "Test Name"(u16 0) -> ()
                n126 = property on="Progress" class="Clust (strict)"("Visible"=FALSE) -> ()  [unwired: 2 in, 2 out]
              }
            }
            n127 = property on="Test Tree" class="Tree (strict)"("Active Item Row Number"=w234, "ActiveColNum"=w234, "CellBG"=w231, "Active Item Row Number"=-1 ("Active Item:Row Number"), "CellBG"=u32 5789784 ("Color Box")) -> ()  [unwired: 2 in, 2 out]
          }
          frame "Variables" {
            w246 = string[] ["CameraPublisher", "Usage", "DB"]  # Items to initially close
            n128 = First Call?() -> (First Call?: T/F=w247:bool)
            n129 = control-ref of="Tree"() -> (w248:refnum<vi>)
            n130 = Select(t=w246, s=w247, f=string[] []) -> (s? t:f=w244:string[])
            n131 = call <vilib>:"NT Read and Format Entries as Tree.vi"("Tags to  Close"=w244, "Tree Refnum"=w248) -> ()  [unwired: 8 in, 2 out]
          }
          frame "Commands" {
            w257 = u32 5789784 ("Color Box")
            w258 = T32 {"Row"=-1, "Column"=-2} ("Active Cell:Active Cell")
            w260 = T32 {"Row"=-2, "Column"=-2} ("Active Cell:Active Cell")
            n132 = Index Array(array=w261, index=w255) -> (element=w259:u32)
            n133 = Index Array(array=w256, index=w255) -> (element=w254:T31)
            n134 = Unbundle(w254) -> ("Operation"=w253:enum16{"Update", "Clear"})  [unwired: 1 out]
            n135 = local read "Command Selection"() -> (w252:i32)
            n136 = property on="Command Selection" class="MCListbox (strict)"("ActiveCell"=w260, "CellBG"=w259, "ActiveCell"=w258, "CellBG"=w257) -> ()  [unwired: 2 in, 2 out]
            n137 = call <vilib>:"WPI_DashboardUpdate RPC Info.vi"("Operation"=w253) -> ("update"=w251:bool, "commands"=w250:string[][])  [unwired: 9 in]
            n138 = property on="Command Selection" class="MCListbox (strict)"("ItemNames"=w250) -> ()  [unwired: 2 in, 2 out]
            n139 = property on="Command Params" class="Tbl (strict)"("Active Cell"=w260, "Cell BG Color"=w259, "Active Cell"=w258, "Cell BG Color"=w257) -> ()  [unwired: 2 in, 2 out]
            n140 = call <vilib>:"WPI_DashboardUpdate Command Params.vi"("Update"=w251, "NewVal"=w252, "Commands"=w250, "Param Tbl"=w249) -> ()  [unwired: 7 in, 1 out]
          }
        }
        n141 = call <vilib>:"Connextion Info.vi"() -> ("Connected"=→"NT Connection":bool)  [unwired: 10 in, 1 out]
      }
      event "Test Tree": Value Change {
        # "Show appropriate\ncontrols"
        n142 = event-data() -> ("CtlRef"=w266:refnum<vi>, "NewVal"=w264:string)  [unwired: 1 in]
        n143 = call <vilib>:"WPI_UtilitiesGetTreeIOName.vi"("NewVal"=w264, "TreeControl in"=w266) -> ("I/O Name"=w267:string)  [unwired: 9 in]
        n144 = case shown="\"Camera\"" w267 {
          selector: w267 -> [_ w274 _ w296 w305 _]
          tunnel: w264 -> [_ _ w293 w295 _ w312]
          tunnel: cluster{string[]}[] [{["640x480", "320x240", "160x120"]}, {["Auto", "Fixed indoor", "Fixed outdoor 1", "Fixed outdoor 2", "Fixed fluorescent 1", "Fixed fluorescent 2", "Hold current"]}, {["Auto", "Flicker-free 50 Hz", "Flicker-free 60 Hz", "Hold current"]}, {["None", "Prioritize frame rate", "Prioritize image quality"]}, {["Monochrome", "Color"]}] -> [_ _ _ _ _ w311]
          frame Default {
            w269 = FALSE ("Visible")
            w268 = FALSE ("Visible")
            n145 = property on="Motor" class="Clust (strict)"("Visible"=w268) -> ()  [unwired: 2 in, 2 out]
            n146 = property on="Test Ring" class="Ring (strict)"("Visible"=w268) -> ()  [unwired: 2 in, 2 out]
            n147 = property on="Rev/Fwd" class="Clust (strict)"("Visible"=w269) -> ()  [unwired: 2 in, 2 out]
            n148 = property on="On/Off" class="Bool (strict)"("Visible"=w269) -> ()  [unwired: 2 in, 2 out]
            n149 = property on="Test Slider" class="Slide (strict)"("Visible"=w269) -> ()  [unwired: 2 in, 2 out]
          }
          frame "Analog Out", "Motor", "PWM" {
            w275 = FALSE ("Visible")
            n150 = case shown="\"Analog Out\"" w274 {
              tunnel: [1.0 ("Value") -1.0 ("Value") 0.0 ("Value")] -> w273
              tunnel: [255.0 ("Value") 1.0 ("Value") 5.0 ("Value")] -> w272
              tunnel: [128.0 ("Value") 0.0 ("Value") 0.0 ("Value")] -> w271
              tunnel: [64.0 ("Value") 0.5 ("Value") 1.0 ("Value")] -> w270
              frame "PWM" {
              }
              frame "Motor", Default {
              }
              frame "Analog Out" {
              }
            }
            n151 = property on="Motor" class="Clust (strict)"("Visible"=TRUE) -> ()  [unwired: 2 in, 2 out]
            n152 = property on="Value" class="Slide (strict)"("Value"=w271, "Scale.Minimum"=w273, "Scale.Maximum"=w272, "Scale.Increment"=w270) -> ()  [unwired: 2 in, 2 out]
            n153 = property on="On/Off" class="Bool (strict)"("Visible"=w275) -> ()  [unwired: 2 in, 2 out]
            n154 = property on="Test Slider" class="Slide (strict)"("Visible"=w275) -> ()  [unwired: 2 in, 2 out]
            n155 = property on="Test Ring" class="Ring (strict)"("Visible"=w275) -> ()  [unwired: 2 in, 2 out]
            n156 = property on="Rev/Fwd" class="Clust (strict)"("Visible"=w275) -> ()  [unwired: 2 in, 2 out]
          }
          frame "Servo" {
            w291 = FALSE ("Visible")
            n157 = call <vilib>:"NT Read Number.vi"("Name"=w293) -> ("Numeric"=w292:dbl)  [unwired: 9 in, 1 out]
            n158 = property on="Test Slider" class="Slide (strict)"("Visible"=TRUE, "Scale.Maximum"=170.0 ("Scale.Range:Maximum")) -> ()  [unwired: 2 in, 2 out]
            n159 = local write "Test Slider"(w292) -> ()
            n160 = property on="Motor" class="Clust (strict)"("Visible"=w291) -> ()  [unwired: 2 in, 2 out]
            n161 = property on="Rev/Fwd" class="Clust (strict)"("Visible"=w291) -> ()  [unwired: 2 in, 2 out]
            n162 = property on="On/Off" class="Bool (strict)"("Visible"=w291) -> ()  [unwired: 2 in, 2 out]
            n163 = property on="Test Ring" class="Ring (strict)"("Visible"=w291) -> ()  [unwired: 2 in, 2 out]
          }
          frame "Relay", "Solenoid" {
            w294 = FALSE ("Visible")
            n164 = property on="Motor" class="Clust (strict)"("Visible"=w294) -> ()  [unwired: 2 in, 2 out]
            n165 = property on="Test Slider" class="Slide (strict)"("Visible"=w294) -> ()  [unwired: 2 in, 2 out]
            n166 = Search and Replace String(input string=w295, search string="/Value  **", replace string="/Direction") -> (result string=w301:string)  [unwired: 5 in, 3 out]
            n167 = property on="Test Ring" class="Ring (strict)"("Visible"=w294) -> ()  [unwired: 2 in, 2 out]
            n168 = call <vilib>:"NT Read String.vi"("Name"=w301) -> ("String"=w299:string)  [unwired: 9 in, 1 out]
            n169 = Equal?(x="Both directions", y=w299) -> (x = y?=w297:bool)
            n170 = Not(x=w297) -> (.not. x?=w298:bool)
            n171 = property on="Rev/Fwd" class="Clust (strict)"("Visible"=w297) -> ()  [unwired: 2 in, 2 out]
            n172 = property on="On/Off" class="Bool (strict)"("Visible"=w298, "Caption.Text"=w296) -> ()  [unwired: 2 in, 2 out]
          }
          frame "Compressor", "Digital Out" {
            w304 = FALSE ("Visible")
            # "Get direction and finish"
            n173 = property on="Motor" class="Clust (strict)"("Visible"=w304) -> ()  [unwired: 2 in, 2 out]
            n174 = property on="Test Slider" class="Slide (strict)"("Visible"=w304) -> ()  [unwired: 2 in, 2 out]
            n175 = property on="Test Ring" class="Ring (strict)"("Visible"=w304) -> ()  [unwired: 2 in, 2 out]
            n176 = property on="On/Off" class="Bool (strict)"("Visible"=TRUE, "Caption.Text"=w305) -> ()  [unwired: 2 in, 2 out]
            n177 = property on="Rev/Fwd" class="Clust (strict)"("Visible"=FALSE) -> ()  [unwired: 2 in, 2 out]
          }
          frame "Camera" {
            n178 = call <vilib>:"Get Last Path Segment.vi"("String in"=w312) -> ("String out"=w313:string)  [unwired: 10 in]
            n179 = property on="On/Off" class="Bool (strict)"("Visible"=FALSE) -> ()  [unwired: 2 in, 2 out]
            n180 = property on="Motor" class="Clust (strict)"("Visible"=FALSE) -> ()  [unwired: 2 in, 2 out]
            n181 = property on="Rev/Fwd" class="Clust (strict)"("Visible"=FALSE) -> ()  [unwired: 2 in, 2 out]
            n182 = case shown="\"White Balance  **\"" w313 {
              tunnel: w312 -> [w319 w328 w337 w346 w355 _ w361]
              tunnel: w311 -> [w317 w325 w334 w343 w352 _ _]
              frame "Size  **" {
                n183 = Index Array(array=w317) -> (element=w316:cluster{string[]})  [unwired: 1 in]
                n184 = call <vilib>:"NT Read String.vi"("Name"=w319) -> ("String"=w318:string)  [unwired: 9 in, 1 out]
                n185 = Unbundle(w316) -> (w314:string[])
                n186 = Match First String(2:w314, 3:w318) -> (0:w315:i32)  [unwired: 1 out]
                n187 = property on="Test Ring" class="Ring (strict)"("Value"=w315, "Strings []"=w314) -> ()  [unwired: 2 in, 2 out]
                n188 = property on="Test Ring" class="Ring (strict)"("Visible"=TRUE) -> ()  [unwired: 2 in, 2 out]
                n189 = property on="Test Slider" class="Slide (strict)"("Visible"=FALSE) -> ()  [unwired: 2 in, 2 out]
              }
              frame "White Balance  **" {
                n190 = Index Array(array=w325, index=1) -> (element=w326:cluster{string[]})
                n191 = call <vilib>:"NT Read String.vi"("Name"=w328) -> ("String"=w327:string)  [unwired: 9 in, 1 out]
                n192 = Unbundle(w326) -> (w323:string[])
                n193 = Match First String(2:w323, 3:w327) -> (0:w322:i32)  [unwired: 1 out]
                n194 = property on="Test Ring" class="Ring (strict)"("Value"=w322, "Strings []"=w323) -> ()  [unwired: 2 in, 2 out]
                n195 = property on="Test Ring" class="Ring (strict)"("Visible"=TRUE) -> ()  [unwired: 2 in, 2 out]
                n196 = property on="Test Slider" class="Slide (strict)"("Visible"=FALSE) -> ()  [unwired: 2 in, 2 out]
              }
              frame "Exposure  **" {
                n197 = Index Array(array=w334, index=2) -> (element=w335:cluster{string[]})
                n198 = call <vilib>:"NT Read String.vi"("Name"=w337) -> ("String"=w336:string)  [unwired: 9 in, 1 out]
                n199 = Unbundle(w335) -> (w331:string[])
                n200 = Match First String(2:w331, 3:w336) -> (0:w332:i32)  [unwired: 1 out]
                n201 = property on="Test Ring" class="Ring (strict)"("Value"=w332, "Strings []"=w331) -> ()  [unwired: 2 in, 2 out]
                n202 = property on="Test Ring" class="Ring (strict)"("Visible"=TRUE) -> ()  [unwired: 2 in, 2 out]
                n203 = property on="Test Slider" class="Slide (strict)"("Visible"=FALSE) -> ()  [unwired: 2 in, 2 out]
              }
              frame "Exposure Priority  **" {
                n204 = Index Array(array=w343, index=3) -> (element=w344:cluster{string[]})
                n205 = call <vilib>:"NT Read String.vi"("Name"=w346) -> ("String"=w345:string)  [unwired: 9 in, 1 out]
                n206 = Unbundle(w344) -> (w340:string[])
                n207 = Match First String(2:w340, 3:w345) -> (0:w341:i32)  [unwired: 1 out]
                n208 = property on="Test Ring" class="Ring (strict)"("Value"=w341, "Strings []"=w340) -> ()  [unwired: 2 in, 2 out]
                n209 = property on="Test Ring" class="Ring (strict)"("Visible"=TRUE) -> ()  [unwired: 2 in, 2 out]
                n210 = property on="Test Slider" class="Slide (strict)"("Visible"=FALSE) -> ()  [unwired: 2 in, 2 out]
              }
              frame "Color Enable  **" {
                n211 = Index Array(array=w352, index=4) -> (element=w353:cluster{string[]})
                n212 = call <vilib>:"NT Read String.vi"("Name"=w355) -> ("String"=w354:string)  [unwired: 9 in, 1 out]
                n213 = Unbundle(w353) -> (w349:string[])
                n214 = Match First String(2:w349, 3:w354) -> (0:w350:i32)  [unwired: 1 out]
                n215 = property on="Test Ring" class="Ring (strict)"("Value"=w350, "Strings []"=w349) -> ()  [unwired: 2 in, 2 out]
                n216 = property on="Test Ring" class="Ring (strict)"("Visible"=TRUE) -> ()  [unwired: 2 in, 2 out]
                n217 = property on="Test Slider" class="Slide (strict)"("Visible"=FALSE) -> ()  [unwired: 2 in, 2 out]
              }
              frame Default {
                n218 = property on="Test Ring" class="Ring (strict)"("Visible"=FALSE) -> ()  [unwired: 2 in, 2 out]
                n219 = property on="Test Slider" class="Slide (strict)"("Visible"=FALSE) -> ()  [unwired: 2 in, 2 out]
              }
              frame "Brightness  **", "Color Level  **", "Compression  **", "FPS  **", "Sharpness  **" {
                n220 = call <vilib>:"NT Read Number.vi"("Name"=w361) -> ("Numeric"=w360:dbl)  [unwired: 9 in, 1 out]
                n221 = local write "Test Slider"(w360) -> ()
                n222 = property on="Test Slider" class="Slide (strict)"("Visible"=TRUE, "Scale.Maximum"=100.0 ("Scale.Range:Maximum")) -> ()  [unwired: 2 in, 2 out]
                n223 = property on="Test Ring" class="Ring (strict)"("Visible"=FALSE) -> ()  [unwired: 2 in, 2 out]
              }
            }
          }
        }
        n224 = property on="Progress" class="Clust (strict)"("Visible"=FALSE) -> ()  [unwired: 2 in, 2 out]
      }
      event "Test Name": Mouse Enter {
        # "Populate the ring with the list of tests"
        n225 = event-data() -> ()  [unwired: 1 in, 1 out]
        n226 = call <vilib>:"NT Read String Array.vi"("Name"="TestMode/TestList") -> ("String Array"=w369:string[])  [unwired: 9 in, 1 out]
        n227 = Build Array (concatenate)("Select the test to run...", w369) -> (w368:string[])
        n228 = property on="Test Name" class="Ring (strict)"("Strings []"=w368) -> ()  [unwired: 2 in, 2 out]
      }
      event "Test Name": Value Change {
        w371 = FALSE ("Visible")
        # "Tell the robot the test name to run"
        n229 = event-data() -> ("NewVal"=w375:u16)  [unwired: 1 in]
        n230 = property on="Test Name" class="Ring (strict)"() -> ("Strings []"=w376:string[])  [unwired: 2 in, 2 out]
        n231 = local write "Progress"(T7 {"Test Progress"=0, "Test Progress Text"=""} ("Progress")) -> ()
        n232 = Index Array(array=w376, index=w375) -> (element=w374:string)
        n233 = call <vilib>:"NT Write String.vi"("String"=w374, "Name"="TestMode/TestName") -> ()  [unwired: 9 in, 1 out]
        n234 = property on="Progress" class="Clust (strict)"("Visible"=TRUE) -> ()  [unwired: 2 in, 2 out]
        n235 = property on="Motor" class="Clust (strict)"("Visible"=w371) -> ()  [unwired: 2 in, 2 out]
        n236 = property on="Test Slider" class="Slide (strict)"("Visible"=w371) -> ()  [unwired: 2 in, 2 out]
        n237 = property on="On/Off" class="Bool (strict)"("Visible"=w371) -> ()  [unwired: 2 in, 2 out]
        n238 = property on="Rev/Fwd" class="Clust (strict)"("Visible"=w371) -> ()  [unwired: 2 in, 2 out]
        n239 = property on="Test Ring" class="Ring (strict)"("Visible"=w371) -> ()  [unwired: 2 in, 2 out]
      }
      event "Select Auto": Mouse Enter {
        # "Populate the combo box with the list of autonomous options"
        n240 = event-data() -> ()  [unwired: 1 in, 1 out]
        n241 = call <vilib>:"NT Read String Array.vi"("Name"="Auto List") -> ("String Array"=w378:string[])  [unwired: 9 in, 1 out]
        n242 = property on="Select Auto" class="CmbBox"("Strings[]"=w378) -> ()  [unwired: 2 in, 2 out]
      }
      event "Select Auto": Value Change {
        # "User modified the Auto Selection. Write to NT variable so robot knows."
        n243 = event-data() -> ("NewVal"=w381:string)  [unwired: 1 in]
        n244 = call <vilib>:"NT Write String.vi"("String"=w381, "Name"="Auto Selector") -> ()  [unwired: 9 in, 1 out]
      }
      event "Command Selection": Value Change {
        # "Get the params and show in table"
        n245 = event-data() -> ("NewVal"=w387:i32)  [unwired: 1 in]
        n246 = property on="Command Selection" class="MCListbox (strict)"() -> ("ItemNames"=w385:string[][])  [unwired: 2 in, 2 out]
        n247 = call <vilib>:"WPI_DashboardUpdate Command Params.vi"("NewVal"=w387, "Commands"=w385, "Param Tbl"=w386) -> ()  [unwired: 8 in, 1 out]
      }
      event "Execute Command": Value Change {
        # "Started one, Unique ID holds\nresponse"
        n248 = event-data() -> ()  [unwired: 1 in, 1 out]
        n249 = property on="Command Selection" class="MCListbox (strict)"() -> ("ItemNames"=w398:string[][])  [unwired: 2 in, 2 out]
        n250 = Index Array(array=w398, index (row)="Command Selection", index (col)=0) -> (element=w396:string)
        n251 = call <vilib>:"Invoke Commands.vi"("Command Params"="Command Params", "Function Name"=w396) -> ("Params"=w392:u8, "Started"=w391:bool)  [unwired: 7 in, 1 out]
        n252 = Array Subset(array="Command Params", length (row)=w392) -> (w393:string[][])  [unwired: 3 in]
        n253 = Select(t="Executing" ("Cmd Status"), s=w391, f="" ("Cmd Status")) -> (s? t:f=→"Cmd Status":string)
      }
      event "Command Selection": Double Click {
        n254 = event-data() -> ("Row"=w406:i32)  [unwired: 1 in]
        n255 = local read "Command Params"() -> (w405:string[][])
        n256 = property on="Command Selection" class="MCListbox (strict)"() -> ("ItemNames"=w409:string[][])  [unwired: 2 in, 2 out]
        n257 = Index Array(array=w409, index (row)=w406, index (col)=0) -> (element=w407:string)
        n258 = call <vilib>:"Invoke Commands.vi"("Command Params"=w405, "Function Name"=w407) -> ("Params"=w404:u8, "Started"=w399:bool)  [unwired: 7 in, 1 out]
        n259 = Array Subset(array=w405, length (row)=w404) -> (w403:string[][])  [unwired: 3 in]
        n260 = Select(t="Executing" ("Cmd Status"), s=w399, f="" ("Cmd Status")) -> (s? t:f=w400:string)
        n261 = local write "Cmd Status"(w400) -> ()
      }
      event "CheckList": Double Click {
        # "Shift clears all"
        # "Update symbols on the listbox"
        n262 = event-data() -> ("PlatMods.Shift"=w411:bool, "Row"=w413:i32)  [unwired: 1 in]
        n263 = case shown="True" w411 {
          tunnel: w413 -> [w417 _]
          tunnel: 1 -> [w416 _]
          frame False {
            n264 = property on="CheckList" class="LstBox (strict)"() -> ("Item Symbols"=w415:i32[])  [unwired: 2 in, 2 out]
            n265 = Replace Array Subset(array=w415, new element=w416, index=w417) -> (w414:i32[])
            n266 = property on="CheckList" class="LstBox (strict)"("Item Symbols"=w414) -> ()  [unwired: 2 in, 2 out]
          }
          frame True {
            w418 = 0 ("Top Row")
            n267 = property on="CheckList" class="LstBox (strict)"() -> ("Number of Rows"=w420:u32)  [unwired: 2 in, 2 out]
            n268 = Initialize Array(0, w420) -> (w419:i32[])
            n269 = property on="CheckList" class="LstBox (strict)"("Top Row"=w418, "Value"=w418, "Item Symbols"=w419) -> ()  [unwired: 2 in, 2 out]
          }
        }
      }
      event "CheckList": Key Down {
        # "Update symbols on the listbox\nLeft and right keys check and uncheck"
        n270 = event-data() -> ("VKey"=w424:T29)  [unwired: 1 in]
        n271 = case shown="\"Left\", \"Right\"" w424 {
          selector: w424 -> [w429 _]
          tunnel: eventvkey."Left" ("VKey") -> [w427 _]
          frame "Left", "Right" {
            n272 = Equal?(x=w427, y=w429) -> (x = y?=w428:bool)
            n273 = Select(t=0, s=w428, f=1) -> (s? t:f=w430:i32)
            n274 = property on="CheckList" class="LstBox (strict)"() -> ("Item Symbols"=w433:i32[])  [unwired: 2 in, 2 out]
            n275 = Replace Array Subset(array=w433, new element=w430, index="CheckList") -> (w432:i32[])
            n276 = property on="CheckList" class="LstBox (strict)"("Item Symbols"=w432) -> ()  [unwired: 2 in, 2 out]
          }
          frame Default {
          }
        }
      }
      event "Motor.Enable": Value Change {
        # "When the test mode otor enable helper is set, update that\ntree row item's value"
        n277 = event-data() -> ("NewVal"=w439:bool)  [unwired: 1 in]
        n278 = Unbundle("Motor") -> ("Value"=w438:dbl)  [unwired: 1 out]
        n279 = Select(t=w438, s=w439, f=0.0) -> (s? t:f=w436:dbl)
        n280 = call <vilib>:"NT Write Number.vi"("Numeric"=w436, "Name"=w435) -> ()  [unwired: 9 in, 1 out]
      }
      event "Test Slider": Value Change {
        # "When the test mode slider helper is set, update that\ntree row item's value"
        n281 = event-data() -> ("NewVal"=w442:dbl)  [unwired: 1 in]
        n282 = call <vilib>:"NT Write Number.vi"("Numeric"=w442, "Name"=w443) -> ()  [unwired: 9 in, 1 out]
      }
      event "On/Off": Value Change {
        # "When the test mode on/off helper value is set, update that\ntree row item's value"
        n283 = event-data() -> ("NewVal"=w447:bool)  [unwired: 1 in]
        n284 = Boolean To (0,1)(Boolean=w447) -> (0, 1=w446:i16)
        n285 = call <vilib>:"NT Write Number.vi"("Numeric"=w446, "Name"=w445) -> ()  [unwired: 9 in, 1 out]
      }
      event "Rev/Fwd": Value Change {
        # "When the test mode helper value for relays is set, update that\ntree row item's value"
        n286 = event-data() -> ("NewVal.Forward"=w455:bool, "NewVal.Reverse"=w454:bool)  [unwired: 1 in]
        n287 = Boolean To (0,1)(Boolean=w455) -> (0, 1=w451:i16)
        n288 = Boolean To (0,1)(Boolean=w454) -> (0, 1=w453:i16)
        n289 = Negate(x=w453) -> (-x=w452:i16)
        n290 = Add(x=w451, y=w452) -> (x+y=w450:i16)
        n291 = call <vilib>:"NT Write Number.vi"("Numeric"=w450, "Name"=w449) -> ()  [unwired: 9 in, 1 out]
      }
      event "Test Ring": Value Change {
        # "When a test mode helper value is selected from the ring,\nset the tree item's variable to the string value"
        n292 = event-data() -> ("NewVal"=w459:u16)  [unwired: 1 in]
        n293 = property on="Test Ring" class="Ring (strict)"() -> ("Strings []"=w460:string[])  [unwired: 2 in, 2 out]
        n294 = Index Array(array=w460, index=w459) -> (element=w458:string)
        n295 = call <vilib>:"NT Write String.vi"("String"=w458, "Name"=w457) -> ()  [unwired: 9 in, 1 out]
      }
      event "Rec Mode": Value Change {
        # "Update globals for recording mode and path to read log from.\nClear when logging and let NetworkTables set path for vision to\nuse."
        n296 = event-data() -> ("NewVal"=w471:enum32{"Stop", "Record", "Playback"})  [unwired: 1 in]
        n297 = global write "WPI_DashboardLogging Global.vi" "Logging Filename"(path "") -> ()
        n298 = global write "WPI_DashboardLogging Global.vi" "Recording"(w471) -> ()
        n299 = case shown="\"Playback\"" w471 {
          tunnel: w470 -> [_ w473 w482]
          tunnel: [_ _ w481] -> w468
          tunnel: [_ _ w480] -> _
          tunnel: w466 -> [_ _ w478]
          tunnel: cluster{i32, i32} {-250, 170} -> [_ _ w477]
          tunnel: [_ _ T30 {"Image Size"=TRUE, "Image Type"=TRUE, "Pixel Value"=TRUE, "ROI Information"=TRUE, "Zoom Factor"=FALSE} ("Image Information Shown:All Elements")] -> w461
          tunnel: [_ _ TRUE ("Zoom Factor")] -> w462
          tunnel: w464 -> [_ _ w474]
          frame Default {
          }
          frame "Stop", "Record" {
            # "Place Window too"
            n300 = invoke class="VI" method="FP.Close"(reference=w473) -> (reference out=w472:refnum<vi>)  [unwired: 2 in, 2 out]
            n301 = invoke class="VI" method="Abort VI"(reference=w472) -> ()  [unwired: 2 in, 3 out]
          }
          frame "Playback" {
            n302 = call "Open Playback Panel.vi"("Offset"=w477, "DB VI Ref"=w478, "Playback in"=w482) -> ("Playback out"=w479:refnum<vi>)  [unwired: 8 in]
            n303 = register-events(w479, w474) -> (reference out=w481:refnum<event-registration>, error out=w480:errorcluster)  [unwired: 2 in]
          }
        }
        n304 = property on="Camera Image Right" class="ImageControl"("Image Information Shown"=w461, "Image Information Visible"=w462) -> ()  [unwired: 2 in, 2 out]
        n305 = property on="Camera Image" class="ImageControl"("Image Information Shown"=w461, "Image Information Visible"=w462) -> ()  [unwired: 2 in, 2 out]
        n306 = call <vilib>:"WPI_DashboardNT Log FieldName Cache.vi"("Operation"=enum16{"Lookup/Add", "Index", "Clear"}."Clear") -> ()  [unwired: 8 in, 3 out]
      }
      event Panel Close {
        w484 = enum32{"Stop", "Record", "Playback"}."Stop" ("Rec Mode")
        # "Playback window has been closed, abort"
        n307 = event-data() -> ()  [unwired: 1 in, 4 out]
        n308 = local write "Rec Mode"(w484) -> ()
        n309 = global write "WPI_DashboardLogging Global.vi" "Recording"(w484) -> ()
      }
      event Panel Close {
        # "Abort playback window and ourself"
        n310 = event-data() -> ()  [unwired: 1 in, 4 out]
        n311 = invoke class="VI" method="FP.Close"(reference=w488) -> (reference out=w487:refnum<vi>)  [unwired: 2 in, 2 out]
        n312 = invoke class="VI" method="Abort VI"(reference=w487) -> (error out=w486:errorcluster)  [unwired: 2 in, 2 out]
        n313 = invoke class="VI" method="Abort VI"(error in=w486) -> ()  [unwired: 2 in, 3 out]
      }
      event User Event {
        n314 = event-data() -> ("IDs"=w495:cluster{"RPC field ID":u16, "Unique ID":u16}, "String"=w494:string)  [unwired: 1 in]
        n315 = Bundle("IDs"=w495, "String"=w494) -> (w493:T10)  [unwired: 1 in]
        n316 = call <vilib>:"Retrieve RPC Response.vi"("RPC Response"=w493) -> ("Output"=w491:string[][])  [unwired: 10 in]
        n317 = Build Array (concatenate)(w489, w491) -> (w490:string[][])
        n318 = local write "Command Params"(w490) -> ()
        n319 = local write "Cmd Status"("" ("Cmd Status")) -> ()
      }
      event "Tree": Double Click {
        n320 = event-data() -> ("PlatMods"=w501:T33, "Tag"=w498:string)  [unwired: 1 in]
        n321 = Unbundle(w501) -> ("Shift"=w500:bool)  [unwired: 4 out]
        n322 = String Subset(string=w498, length (rest)=1 ("length (rest)")) -> (substring=w497:string)  [unwired: 1 in]
        n323 = Not(x=w500) -> (.not. x?=w499:bool)
        n324 = case shown="\"/\"" w497 {
          tunnel: w498 -> [_ w504]
          tunnel: w499 -> [_ w503]
          frame Default {
          }
          frame "/" {
            n325 = call <vilib>:"NT Update Persistence.vi"("Persistence"=w503, "Name"=w504) -> ()  [unwired: 9 in, 1 out]
          }
        }
      }
    }
  }
  n326 = while {
    tunnel: w65 -> [w506]
    i -> [w509]
    stop <- FALSE stop-if-true
    n327 = Wait (ms)(milliseconds to wait=u32 100) -> ()  [unwired: 1 out]
    n328 = case shown="\"Playback\"" "Rec Mode" {
      tunnel: w509 -> [_ _ w524]
      tunnel: [u32 2829099 ("Base Color") u32 11141120 ("Target Color") w513] -> w505
      frame "Stop", Default {
        # "Reset the color, extra updates don't cost much"
      }
      frame "Record" {
      }
      frame "Playback" {
        # "Playback"
        n329 = Quotient & Remainder(x=w524, y=u32 50 ("milliseconds to wait")) -> (x-y*floor(x/y)=w520:u32)  [unwired: 1 out]
        n330 = Divide(x=w520, y=u32 50 ("milliseconds to wait")) -> (x/y=w517:dbl)
        n331 = Multiply(x=6.283185307179586, y=w517) -> (x*y=w522:dbl)
        n332 = Sine(x=w522) -> (sin(x)=w521:dbl)
        n333 = Absolute Value(x=w521) -> (abs(x)=w514:dbl)
        n334 = call "Interpolate RGB Color.vi"("Proportion"=w514, "Target Color"=u32 30976, "Base Color"=u32 2829099) -> ("Result Color"=w513:u32)  [unwired: 8 in]
      }
    }
    n335 = property class="Pane"(reference=w506, "PaneColor"=w505) -> ()  [unwired: 1 in, 2 out]
  }
  n336 = local write "Dashboard Tab"(T2."Drive" ("Dashboard Tab")) -> ()
  n337 = property on="On/Off" class="Bool (strict)"("Visible"=w36) -> ()  [unwired: 2 in, 2 out]
  n338 = property on="Motor" class="Clust (strict)"("Visible"=w36) -> ()  [unwired: 2 in, 2 out]
  n339 = property on="Progress" class="Clust (strict)"("Visible"=w36) -> ()  [unwired: 2 in, 2 out]
  n340 = property on="Test Ring" class="Ring (strict)"("Visible"=w36) -> ()  [unwired: 2 in, 2 out]
  n341 = property on="Rev/Fwd" class="Clust (strict)"("Visible"=w36) -> ()  [unwired: 2 in, 2 out]
  n342 = while {
    tunnel: u16 1741 ("timeout ms (25000)") -> [w526]
    stop <- FALSE stop-if-true
    n343 = TCP Create Listener(10:w526) -> (0:w525:errorcluster, 3:w527:refnum<k5>)  [unwired: 4 in, 1 out]
    n344 = case shown="No Error" w525 {
      selector: w525 -> [w529 _]
      tunnel: w527 -> [w530 _]
      frame No Error {
        n345 = while {
          tunnel: w530 -> [w533]
          tunnel: w529 -> [w532]
          stop <- FALSE stop-if-true
          n346 = TCP Wait On Listener(8:w532, 11:w533) -> (0:w534:errorcluster, 4:w535:refnum<k5>)  [unwired: 2 in, 3 out]
          n347 = local write "TCP"(w535) -> ()
          n348 = case shown="No Error" w534 {
            frame No Error {
            }
            frame Error {
              n349 = Wait (ms)(milliseconds to wait=u32 1000) -> ()  [unwired: 1 out]
            }
          }
        }
      }
      frame Error {
        n350 = Wait (ms)(milliseconds to wait=u32 1000) -> ()  [unwired: 1 out]
      }
    }
  }
  n351 = local write "Command Selection"(u16 0 ("milliseconds to wait")) -> ()
  n352 = local write "Command Params"(string[][] [] ("Command Params")) -> ()
  n353 = global write "WPI_DashboardLogging Global.vi" "Recording"(w59) -> ()
  n354 = local write "Rec Mode"(w59) -> ()
  n355 = call <vilib>:"NT Write String.vi"("String"="Select Auto", "Name"="Auto Selector") -> ()  [unwired: 9 in, 1 out]
